vi "SolenoidSet.vi"(0 "String":string, 1 "Boolean":bool) -> ()   [LabVIEW 2016]
uses:
  <vilib>/Rock Robotics/WPI/SafetyOutput/WPI_SafetyOutputConfigMenu.ctl
  <vilib>/Rock Robotics/WPI/Solenoid/Deprecated/WPI_SolenoidSetBool.vi
  <vilib>/Rock Robotics/WPI/Solenoid/WPI_SolenoidGetEnum.vi
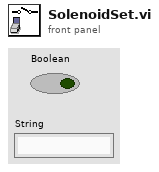
[diagram p1: front panel]
types:
  T1 = typedef "WPI_SafetyOutputConfigMenu.ctl" = enum16{"Enable", "Disable"}
  T2 = typedef "WPI_SolenoidDevRef.ctl" = cluster{"DevStatus":errorcluster, "Pneumatics Control Module":u8, "Forward Solenoid Channel":T3, "Reverse Solenoid Channel":T3}
  T3 = typedef "WPI_SolenoidChannel.ctl" = enum8{"Solenoid 0", "Solenoid 1", "Solenoid 2", "Solenoid 3", "Solenoid 4", "Solenoid 5", "Solenoid 6", "Solenoid 7", "Invalid"}
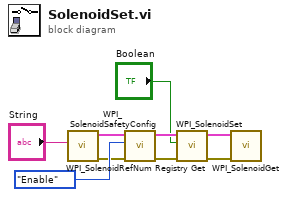
[diagram p0: block diagram]
diagram:
  n1 = call <vilib>:"WPI_SolenoidRefNum Registry Get.vi"("refnum name"="String") -> ("error out"=w5:errorcluster, "SolenoidDevRef"=w7:T2)  [unwired: 9 in]
  n2 = call <vilib>:"WPI_SolenoidSafetyConfig.vi"("error in (no error)"=w5, "mode"=WPI_SafetyOutputConfigMenu."Enable", "SolenoidDevRef"=w7) -> ("error out"=w6:errorcluster, "SolenoidDevRef"=w8:T2)  [unwired: 7 in]
  n3 = call-poly <vilib>:"WPI_SolenoidSet.vi"("error in (no error)"=w6, "Value"="Boolean", "SolenoidDevRef"=w8) -> ("error out"=w3:errorcluster, "SolenoidDevRef"=w4:T2)  [unwired: 7 in]
  n4 = call-poly <vilib>:"WPI_SolenoidGet.vi"("error in (no error)"=w3, "SolenoidDevRef"=w4) -> ()  [unwired: 7 in, 3 out]
